vi "Main.vi"(8 "error in (no error)":errorcluster, 11 "TomoBase in":refnum<class "Tomo.lvclass">) -> (0 "error out":errorcluster, 3 "component":refnum<class "Tomo.lvclass">)   [LabVIEW 2012, in "Tomo.lvclass"]
doc: "Main VI of the component."
uses:
  Tomo.lvclass
  <vilib>/Distrio/Murmex/Murmex/command_enum.ctl
  volume map.ctl
  Tomo.lvclass/Tomo.ctl
  <vilib>/Distrio/Murmex/InitialiseMessage/InitialiseMessage.lvclass
  <vilib>/Distrio/Murmex/TerminateMessage/TerminateMessage.lvclass
  <vilib>/Distrio/Murmex/ConfigureMessage/ConfigureMessage.lvclass
  <vilib>/Distrio/Murmex/Murmex/update_cluster.ctl
  <vilib>/Distrio/Murmex/StopMessage/StopMessage.lvclass
  <vilib>/Distrio/Murmex/GenericMessage/GenericMessage.lvclass
  <vilib>/Distrio/Murmex/Murmex/Set configure at initialise.vi
  <vilib>/Distrio/Murmex/Murmex/Set log reference.vi
  <vilib>/Distrio/Murmex/Murmex/Set VI reference.vi
  <vilib>/Distrio/Murmex/Murmex/Set write log to disk.vi
  <vilib>/Distrio/Murmex/Message/Add or replace parameter.vi
  <vilib>/Distrio/Murmex/Murmex/Murmex.lvclass
  <vilib>/Distrio/Murmex/Message/Message.lvclass
panel:
  in  "Tab Control":T1(tab)
  in  "Volume map":T2
  out "TB":dbl format="%#_2g"
  out "Tomography progress":dbl(slide) scale=0.0..1.0
  in  "experiment name":string
  in  "Z step size":dbl[unit]=1e-06
  in  "X step size":dbl[unit]=0.0005
  in  "Y step size":dbl[unit]=0.0005
  in  "Timelapse stacks":dbl=1.0
  in  "starting angle":dbl[unit]
  in  "button::start":bool
  out "Estimated remaining time":dbl format="- %<%H:%M:%S>t"
  in  "X min":dbl[unit]
  in  "X max":dbl[unit]
  in  "Y min":dbl[unit]
  in  "Y max":dbl[unit]
  in  "Z min":dbl[unit]
  in  "Z max":dbl[unit]
  in  "Pre tomo volume file":path
  in  "Pre tomo binary images path":path
  in  "button::pretomo calc":bool
  in  "Custom volume path":path
  in  "Experimenter email address":string
  in  "Experimenter name":string
  in  "generic command":string
  in  "button::send command":bool
  out "log":string
  in  "ID":string="tomo"
  in  "command":T3
  in  "recipient":string
  in  "button::configure":bool
  in  "button::quit":bool
  in  "terminate?":bool
  # "Tomo\n\nImplemented by:\nLudovico Silvestri\nUniversity of Florence, Italy"
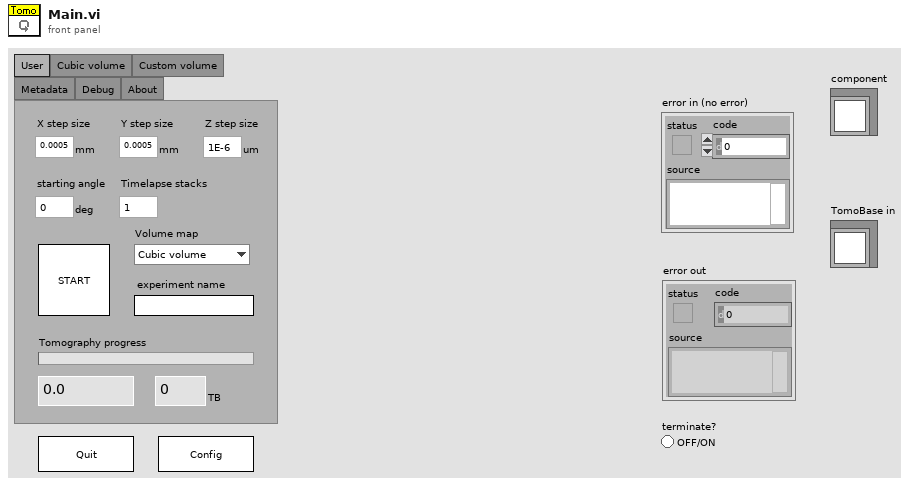
[diagram p1: front panel]
types:
  T1 = enum32{"User", "Cubic volume", "Custom volume", "Metadata", "Debug", "About"}
  T2 = typedef "Tomo.lvclass/volume map.ctl" = enum16{"Cubic volume", "Custom volume", "Self-generate volume", "Time- tomography"}
  T3 = typedef "Murmex.lvlib/Murmex.lvclass/command_enum.ctl" = enum16{"null", "initialise", "reset", "terminate", "acknowledge", "update", "inspect", "inform", "proceed", "start", "stop", "fetch", "configure", "generic"}
  T4 = enum32{"Page Enabled", "Page Disabled", "Page Disabled & Grayed"}
  T5 = typedef "Murmex.lvlib/Murmex.lvclass/update_cluster.ctl" = cluster{"target ID":string, "key chains":string[], "values":variant[]}
  T6 = enum8{"Enabled", "Disabled", "Disabled and Grayed Out"}
  T7 = enum16{"Cubic volume", "Custom volume", "Self-generate volume"}
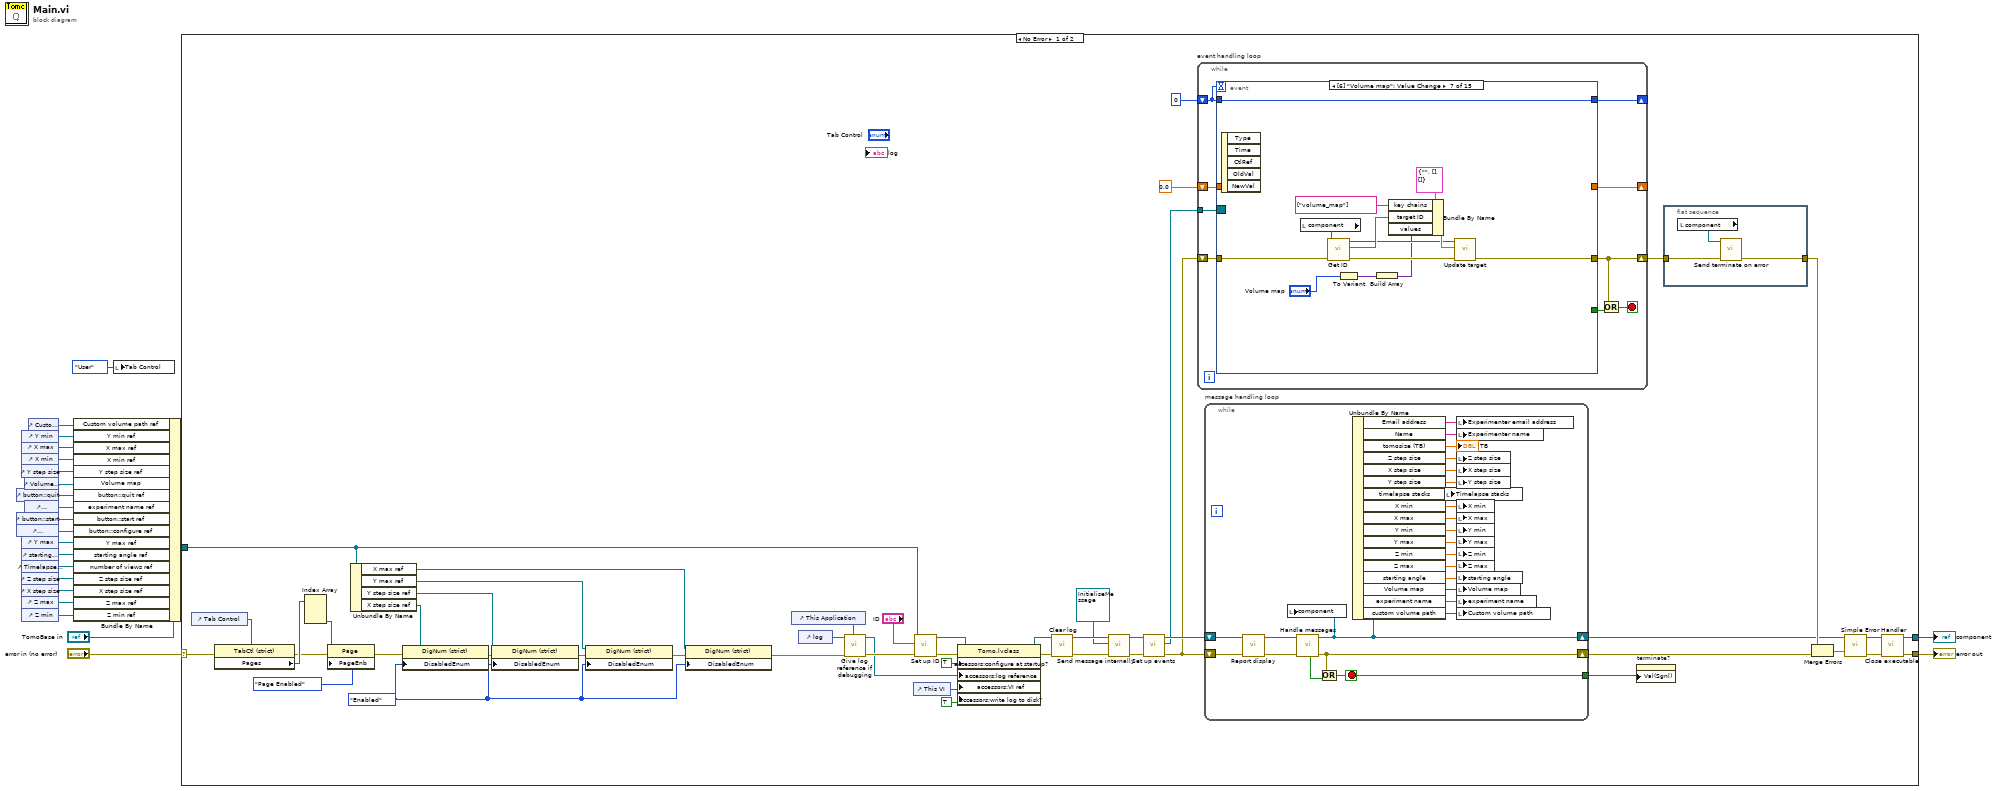
[diagram p0: block diagram]
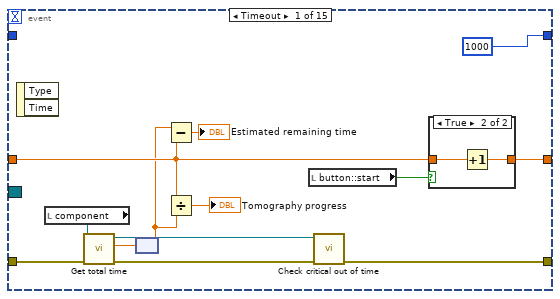
[diagram p2: hidden frame]
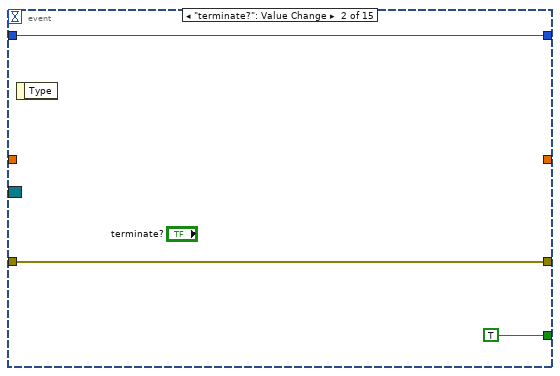
[diagram p4: hidden frame]
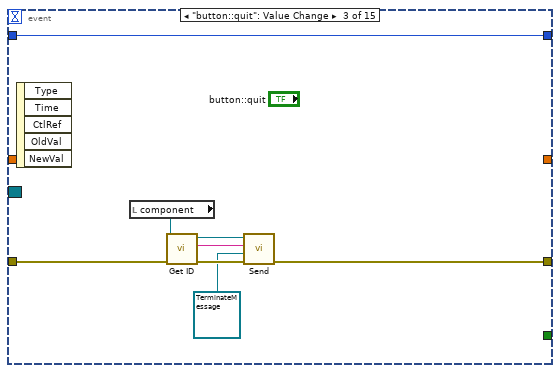
[diagram p5: hidden frame]
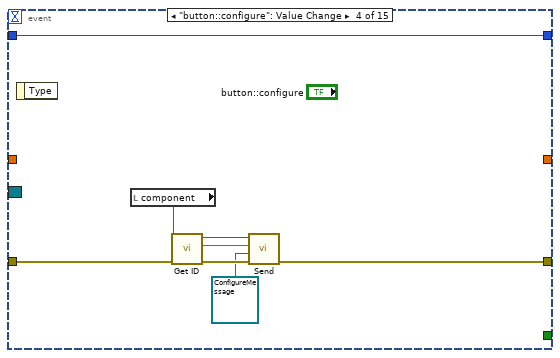
[diagram p6: hidden frame]
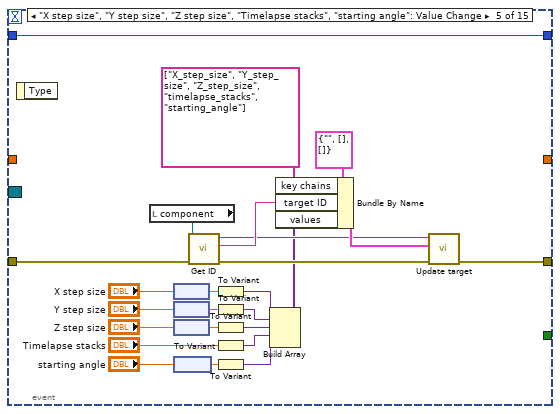
[diagram p7: hidden frame]
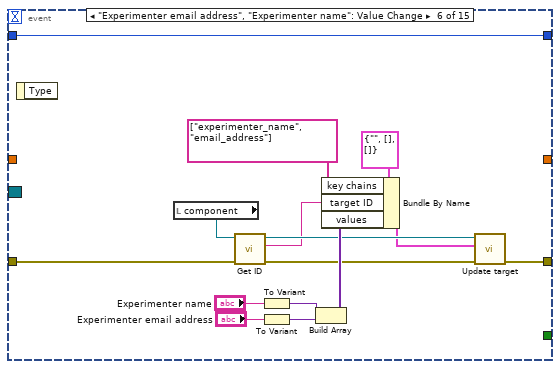
[diagram p8: hidden frame]
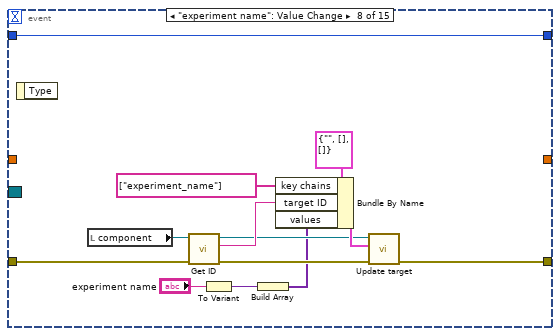
[diagram p9: hidden frame]
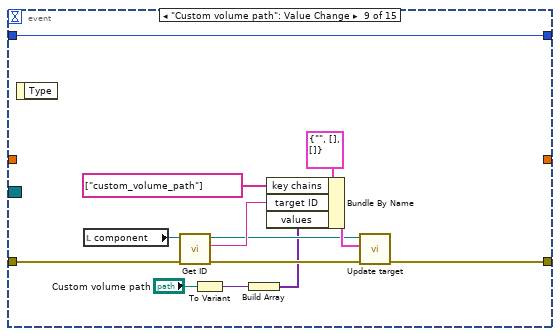
[diagram p10: hidden frame]
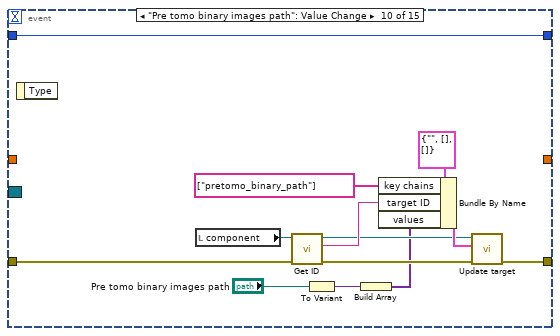
[diagram p11: hidden frame]
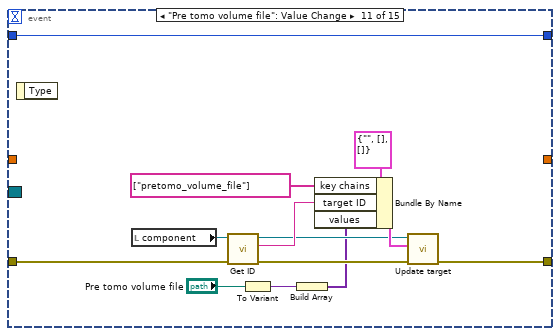
[diagram p12: hidden frame]
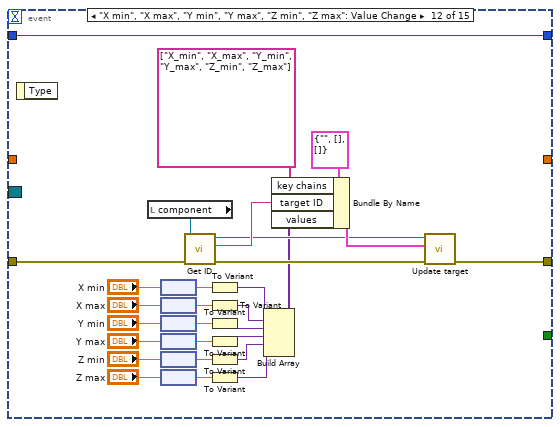
[diagram p13: hidden frame]
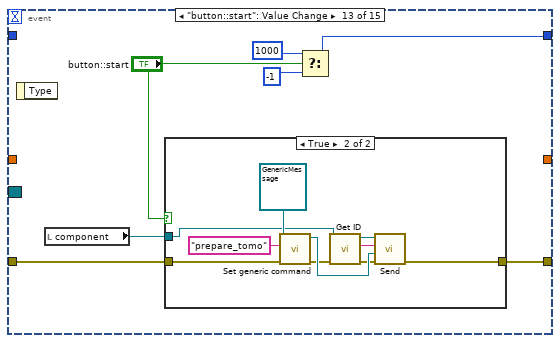
[diagram p14: hidden frame]
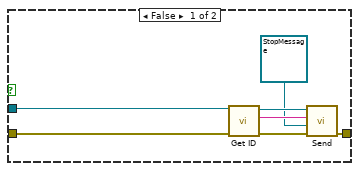
[diagram p15: hidden frame]
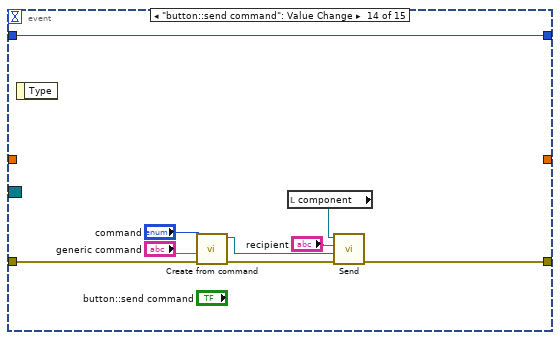
[diagram p16: hidden frame]
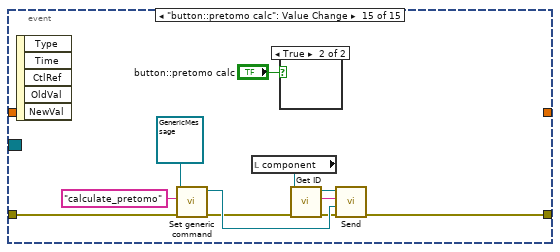
[diagram p17: hidden frame]
diagram:
  n1 = control-ref of="button::quit"() -> (w13:refnum<vi>)
  n2 = control-ref of="button::start"() -> (w11:refnum<vi>)
  n3 = control-ref of="button::configure"() -> (w10:refnum<vi>)
  n4 = control-ref of="Y min"() -> (w17:refnum<vi>)
  n5 = control-ref of="X max"() -> (w16:refnum<vi>)
  n6 = control-ref of="X min"() -> (w15:refnum<vi>)
  n7 = control-ref of="Y step size"() -> (w14:refnum<vi>)
  n8 = control-ref of="Y max"() -> (w9:refnum<vi>)
  n9 = control-ref of="starting angle"() -> (w8:refnum<vi>)
  n10 = control-ref of="Timelapse stacks"() -> (w7:refnum<vi>)
  n11 = control-ref of="Z step size"() -> (w6:refnum<vi>)
  n12 = control-ref of="X step size"() -> (w5:refnum<vi>)
  n13 = control-ref of="Z max"() -> (w4:refnum<vi>)
  n14 = control-ref of="Z min"() -> (w3:refnum<vi>)
  n15 = control-ref of="Volume map"() -> (w1:refnum<vi>)
  n16 = control-ref of="experiment name"() -> (w12:refnum<vi>)
  n17 = control-ref of="Custom volume path"() -> (w18:refnum<vi>)
  n18 = Bundle By Name(cluster="TomoBase in", "Custom volume path ref"=w18, "Y min ref"=w17, "X max ref"=w16, "X min ref"=w15, "Y step size ref"=w14, "Volume map"=w1, "button::quit ref"=w13, "experiment name ref"=w12, "button::start ref"=w11, "button::configure ref"=w10, "Y max ref"=w9, "starting angle ref"=w8, "number of views ref"=w7, "Z step size ref"=w6, "X step size ref"=w5, "Z max ref"=w4, "Z min ref"=w3) -> (w19:refnum<class "Tomo.lvclass">)
  n19 = local write "Tab Control"(T1."User" ("Tab Control")) -> ()
  n20 = case shown="No Error" "error in (no error)" {
    selector: "error in (no error)" -> [w40 w322]
    tunnel: w19 -> [w34 w321]
    tunnel: [w49 w322] -> w22
    tunnel: [w47 w321] -> w21
    frame No Error {
      w24 = T6."Enabled" ("Disabled")
      n21 = control-ref of="Tab Control"() -> (w39:refnum<vi>)
      n22 = property class="TabCtl (strict)"(reference=w39, error in=w40) -> (error out=w37:errorcluster, "Pages"=w38:refnum<vi>[])  [unwired: 1 out]
      n23 = Index Array(array=w38) -> (element #3=w36:refnum<vi>)  [unwired: 3 in, 2 out]
      n24 = property class="Page"(reference=w36, error in=w37, "PageEnb"=T4."Page Enabled" ("Page Enabled State")) -> (error out=w33:errorcluster)  [unwired: 1 out]
      n25 = Unbundle By Name(w34) -> ("X max ref"=w25:refnum<vi>, "Y max ref"=w26:refnum<vi>, "Y step size ref"=w27:refnum<vi>, "X step size ref"=w28:refnum<vi>)
      n26 = property class="DigNum (strict)"(reference=w28, error in=w33, "DisabledEnum"=w24) -> (error out=w32:errorcluster)  [unwired: 1 out]
      n27 = property class="DigNum (strict)"(reference=w27, error in=w32, "DisabledEnum"=w24) -> (error out=w31:errorcluster)  [unwired: 1 out]
      n28 = property class="DigNum (strict)"(reference=w26, error in=w31, "DisabledEnum"=w24) -> (error out=w30:errorcluster)  [unwired: 1 out]
      n29 = property class="DigNum (strict)"(reference=w25, error in=w30, "DisabledEnum"=w24) -> (error out=w29:errorcluster)  [unwired: 1 out]
      n30 = control-ref of="This Application"() -> (w42:refnum<vi>)
      n31 = control-ref of="log"() -> (w44:refnum<vi>)
      n32 = call "Give log reference if debugging.vi"("application ref"=w42, "error in (no error)"=w29, "log reference in"=w44) -> ("error out"=w45:errorcluster, "log reference out"=w43:refnum<vi>)  [unwired: 6 in, 1 out]
      n33 = control-ref of="This VI"() -> (w70:refnum<vi>)
      n34 = call <vilib>:"Set up ID.vi"("error in (no error)"=w45, "component ID"="ID", "MurmexBase in"=w34) -> ("error out"=w69:errorcluster, "MurmexBase out"=w67:refnum<class "Tomo.lvclass">)  [unwired: 6 in, 1 out]
      n35 = property class="Tomo.lvclass"(reference=w67, error in=w69, "accessors:configure at startup?"=TRUE ("configure at startup?"), "accessors:log reference"=w43, "accessors:VI ref"=w70, "accessors:write log to disk?"=TRUE ("write log to disk?")) -> (reference out=w65:refnum<class "Tomo.lvclass">, error out=w66:errorcluster)
      n36 = call <vilib>:"Clear log.vi"("error in (no error)"=w66, "MurmexBase in"=w65) -> ("error out"=w64:errorcluster, "MurmexBase out"=w63:refnum<class "Tomo.lvclass">)  [unwired: 8 in]
      n37 = call <vilib>:"Send message internally.vi"("error in (no error)"=w64, "Message"=refnum<class "InitialiseMessage.lvclass"> refnum ("Message in"), "Murmex in"=w63) -> ("error out"=w61:errorcluster, "Murmex out"=w60:refnum<class "Tomo.lvclass">)  [unwired: 7 in]
      n38 = call <vilib>:"Set up events.vi"("error in (no error)"=w61, "MurmexBase in"=w60) -> ("error out"=w58:errorcluster, "Event Registration Refnum"=w57:refnum<event-registration>, "MurmexBase out"=w59:refnum<class "Tomo.lvclass">)  [unwired: 7 in]
      n39 = while "event handling loop" {
        shift-right: [w78] -> w55
        shift-left: w58 -> [w83]
        tunnel: w57 -> [w82]
        shift-right: [w80] -> _
        shift-left: 0 -> [w81]
        shift-right: [w75] -> _
        shift-left: 0.0 -> [w76]
        stop <- w77 stop-if-true
        n40 = event shown="[6] \"Volume map\": Value Change" {
          selector: w82 -> [_ _ _ _ _ _ _ _ _ _ _ _ _ _ _]
          dyn-events: _ -> [_ _ _ _ _ _ _ _ _ _ _ _ _ _ _]
          timeout: w81 -> [_ _ _ _ _ _ _ _ _ _ _ _ _ _ _]
          tunnel: [w85 w100 w107 w113 w141 w149 w165 w173 w189 w202 w215 w246 w258 w277 w286] -> w78
          tunnel: w83 -> [w96 w100 w109 w114 w139 w148 w167 w176 w188 w201 w214 w244 w257 w283 w287]
          tunnel: w81 -> [_ w99 w102 w110 w122 w143 w164 w172 w184 w198 w211 w230 _ w276 _]
          tunnel: [1000 w99 w102 w110 w122 w143 w164 w172 w184 w198 w211 w230 w252 w276 _] -> w80
          tunnel: [_ TRUE _ _ _ _ _ _ _ _ _ _ _ _ _] -> w79
          tunnel: w76 -> [w94 _ _ _ _ _ _ _ _ _ _ _ _ _ _]
          tunnel: [w93 _ _ _ _ _ _ _ _ _ _ _ _ _ _] -> w75
          event Timeout {
            n41 = event-data() -> ()  [unwired: 1 in, 2 out]
            n42 = local read "component"() -> (w92:refnum<class "Tomo.lvclass">)
            n43 = call-dynamic "Get total time.vi"("error in (no error)"=w96, "Tomo in"=w92) -> ("error out"=w95:errorcluster, "Total time"=w91:dbl[unit], "Tomo out"=w84:refnum<class "Tomo.lvclass">)  [unwired: 7 in]
            n44 = node(w91) -> (w89:dbl)
            n45 = Subtract(x=w89, y=w94) -> (x-y=→"Estimated remaining time":dbl)
            n46 = Divide(x=w94, y=w89) -> (x/y=→"Tomography progress":dbl)
            n47 = local read "button::start"() -> (w86:bool)
            n48 = call-dynamic "Check critical out of time.vi"("error in (no error)"=w95, "Tomo in"=w84) -> ("error out"=w85:errorcluster)  [unwired: 8 in, 1 out]
            n49 = case shown="True" w86 {
              tunnel: w94 -> [_ w98]
              tunnel: [_ w97] -> w93
              frame False {
              }
              frame True {
                n50 = Increment(x=w98) -> (x+1=w97:dbl)
              }
            }
          }
          event "terminate?": Value Change {
            n51 = event-data() -> ()  [unwired: 1 in, 1 out]
          }
          event "button::quit": Value Change {
            n52 = event-data() -> ()  [unwired: 1 in, 5 out]
            n53 = local read "component"() -> (w106:refnum<class "Tomo.lvclass">)
            n54 = call <vilib>:"Get ID.vi"("error in (no error)"=w109, "Murmex in"=w106) -> ("error out"=w108:errorcluster, "component id"=w104:string, "Murmex out"=w105:refnum<class "Tomo.lvclass">)  [unwired: 7 in]
            n55 = call <vilib>:"Send.vi"("error in (no error)"=w108, "Message"=refnum<class "TerminateMessage.lvclass"> refnum ("Distrio Murmex 1.1:TerminateMessage"), "recipient"=w104, "Murmex in"=w105) -> ("error out"=w107:errorcluster)  [unwired: 6 in, 1 out]
          }
          event "button::configure": Value Change {
            n56 = event-data() -> ()  [unwired: 1 in, 1 out]
            n57 = local read "component"() -> (w112:refnum<class "Tomo.lvclass">)
            n58 = call <vilib>:"Get ID.vi"("error in (no error)"=w114, "Murmex in"=w112) -> ("error out"=w117:errorcluster, "component id"=w115:string, "Murmex out"=w116:refnum<class "Tomo.lvclass">)  [unwired: 7 in]
            n59 = call <vilib>:"Send.vi"("error in (no error)"=w117, "Message"=refnum<class "ConfigureMessage.lvclass"> refnum ("Distrio Murmex 1.1:ConfigureMessage"), "recipient"=w115, "Murmex in"=w116) -> ("error out"=w113:errorcluster)  [unwired: 6 in, 1 out]
          }
          event "X step size", "Y step size", "Z step size", "Timelapse stacks", "starting angle": Value Change {
            n60 = event-data() -> ()  [unwired: 1 in, 1 out]
            n61 = local read "component"() -> (w137:refnum<class "Tomo.lvclass">)
            n62 = node("X step size") -> (w121:dbl)
            n63 = node("Y step size") -> (w120:dbl)
            n64 = node("Z step size") -> (w119:dbl)
            n65 = node("starting angle") -> (w118:dbl)
            n66 = call <vilib>:"Get ID.vi"("error in (no error)"=w139, "Murmex in"=w137) -> ("error out"=w140:errorcluster, "component id"=w138:string, "Murmex out"=w135:refnum<class "Tomo.lvclass">)  [unwired: 7 in]
            n67 = To Variant(anything=w121) -> (Variant=w125:variant)
            n68 = To Variant(anything=w120) -> (Variant=w126:variant)
            n69 = To Variant(anything=w119) -> (Variant=w129:variant)
            n70 = To Variant(anything="Timelapse stacks") -> (Variant=w128:variant)
            n71 = To Variant(anything=w118) -> (Variant=w127:variant)
            n72 = Build Array(w125, w126, w129, w128, w127) -> (w124:variant[])
            n73 = Bundle By Name(cluster=T5 {"target ID"="", "key chains"=[], "values"=[]} ("update cluster"), "key chains"=string[] ["X_step_size", "Y_step_size", "Z_step_size", "timelapse_stacks", "starting_angle"], "target ID"=w138, "values"=w124) -> (w136:T5)
            n74 = call <vilib>:"Update target.vi"("error in (no error)"=w140, "update cluster"=w136, "MurmexBase in"=w135) -> ("error out"=w141:errorcluster)  [unwired: 7 in, 1 out]
          }
          event "Experimenter email address", "Experimenter name": Value Change {
            n75 = event-data() -> ()  [unwired: 1 in, 1 out]
            n76 = local read "component"() -> (w144:refnum<class "Tomo.lvclass">)
            n77 = call <vilib>:"Get ID.vi"("error in (no error)"=w148, "Murmex in"=w144) -> ("error out"=w151:errorcluster, "component id"=w152:string, "Murmex out"=w154:refnum<class "Tomo.lvclass">)  [unwired: 7 in]
            n78 = To Variant(anything="Experimenter name") -> (Variant=w156:variant)
            n79 = To Variant(anything="Experimenter email address") -> (Variant=w155:variant)
            n80 = Build Array(w156, w155) -> (w157:variant[])
            n81 = Bundle By Name(cluster=T5 {"target ID"="", "key chains"=[], "values"=[]} ("update cluster"), "key chains"=string[] ["experimenter_name", "email_address"], "target ID"=w152, "values"=w157) -> (w153:T5)
            n82 = call <vilib>:"Update target.vi"("error in (no error)"=w151, "update cluster"=w153, "MurmexBase in"=w154) -> ("error out"=w149:errorcluster)  [unwired: 7 in, 1 out]
          }
          event Value Change {
            n83 = event-data() -> ()  [unwired: 1 in, 5 out]
            n84 = local read "component"() -> (w159:refnum<class "Tomo.lvclass">)
            n85 = call <vilib>:"Get ID.vi"("error in (no error)"=w167, "Murmex in"=w159) -> ("error out"=w166:errorcluster, "component id"=w170:string, "Murmex out"=w168:refnum<class "Tomo.lvclass">)  [unwired: 7 in]
            n86 = To Variant(anything="Volume map") -> (Variant=w163:variant)
            n87 = Build Array(w163) -> (w162:variant[])
            n88 = Bundle By Name(cluster=T5 {"target ID"="", "key chains"=[], "values"=[]} ("update cluster"), "key chains"=string[] ["volume_map"], "target ID"=w170, "values"=w162) -> (w169:T5)
            n89 = call <vilib>:"Update target.vi"("error in (no error)"=w166, "update cluster"=w169, "MurmexBase in"=w168) -> ("error out"=w165:errorcluster)  [unwired: 7 in, 1 out]
          }
          event "experiment name": Value Change {
            n90 = event-data() -> ()  [unwired: 1 in, 1 out]
            n91 = local read "component"() -> (w171:refnum<class "Tomo.lvclass">)
            n92 = call <vilib>:"Get ID.vi"("error in (no error)"=w176, "Murmex in"=w171) -> ("error out"=w180:errorcluster, "component id"=w183:string, "Murmex out"=w181:refnum<class "Tomo.lvclass">)  [unwired: 7 in]
            n93 = To Variant(anything="experiment name") -> (Variant=w179:variant)
            n94 = Build Array(w179) -> (w178:variant[])
            n95 = Bundle By Name(cluster=T5 {"target ID"="", "key chains"=[], "values"=[]} ("update cluster"), "key chains"=string[] ["experiment_name"], "target ID"=w183, "values"=w178) -> (w182:T5)
            n96 = call <vilib>:"Update target.vi"("error in (no error)"=w180, "update cluster"=w182, "MurmexBase in"=w181) -> ("error out"=w173:errorcluster)  [unwired: 7 in, 1 out]
          }
          event "Custom volume path": Value Change {
            n97 = event-data() -> ()  [unwired: 1 in, 1 out]
            n98 = local read "component"() -> (w186:refnum<class "Tomo.lvclass">)
            n99 = call <vilib>:"Get ID.vi"("error in (no error)"=w188, "Murmex in"=w186) -> ("error out"=w193:errorcluster, "component id"=w196:string, "Murmex out"=w194:refnum<class "Tomo.lvclass">)  [unwired: 7 in]
            n100 = To Variant(anything="Custom volume path") -> (Variant=w192:variant)
            n101 = Build Array(w192) -> (w191:variant[])
            n102 = Bundle By Name(cluster=T5 {"target ID"="", "key chains"=[], "values"=[]} ("update cluster"), "key chains"=string[] ["custom_volume_path"], "target ID"=w196, "values"=w191) -> (w195:T5)
            n103 = call <vilib>:"Update target.vi"("error in (no error)"=w193, "update cluster"=w195, "MurmexBase in"=w194) -> ("error out"=w189:errorcluster)  [unwired: 7 in, 1 out]
          }
          event "Pre tomo binary images path": Value Change {
            n104 = event-data() -> ()  [unwired: 1 in, 1 out]
            n105 = local read "component"() -> (w200:refnum<class "Tomo.lvclass">)
            n106 = call <vilib>:"Get ID.vi"("error in (no error)"=w201, "Murmex in"=w200) -> ("error out"=w206:errorcluster, "component id"=w209:string, "Murmex out"=w207:refnum<class "Tomo.lvclass">)  [unwired: 7 in]
            n107 = To Variant(anything="Pre tomo binary images path") -> (Variant=w205:variant)
            n108 = Build Array(w205) -> (w204:variant[])
            n109 = Bundle By Name(cluster=T5 {"target ID"="", "key chains"=[], "values"=[]} ("update cluster"), "key chains"=string[] ["pretomo_binary_path"], "target ID"=w209, "values"=w204) -> (w208:T5)
            n110 = call <vilib>:"Update target.vi"("error in (no error)"=w206, "update cluster"=w208, "MurmexBase in"=w207) -> ("error out"=w202:errorcluster)  [unwired: 7 in, 1 out]
          }
          event "Pre tomo volume file": Value Change {
            n111 = event-data() -> ()  [unwired: 1 in, 1 out]
            n112 = local read "component"() -> (w213:refnum<class "Tomo.lvclass">)
            n113 = call <vilib>:"Get ID.vi"("error in (no error)"=w214, "Murmex in"=w213) -> ("error out"=w219:errorcluster, "component id"=w222:string, "Murmex out"=w220:refnum<class "Tomo.lvclass">)  [unwired: 7 in]
            n114 = To Variant(anything="Pre tomo volume file") -> (Variant=w218:variant)
            n115 = Build Array(w218) -> (w217:variant[])
            n116 = Bundle By Name(cluster=T5 {"target ID"="", "key chains"=[], "values"=[]} ("update cluster"), "key chains"=string[] ["pretomo_volume_file"], "target ID"=w222, "values"=w217) -> (w221:T5)
            n117 = call <vilib>:"Update target.vi"("error in (no error)"=w219, "update cluster"=w221, "MurmexBase in"=w220) -> ("error out"=w215:errorcluster)  [unwired: 7 in, 1 out]
          }
          event "X min", "X max", "Y min", "Y max", "Z min", "Z max": Value Change {
            n118 = event-data() -> ()  [unwired: 1 in, 1 out]
            n119 = local read "component"() -> (w243:refnum<class "Tomo.lvclass">)
            n120 = node("X min") -> (w229:dbl)
            n121 = node("X max") -> (w228:dbl)
            n122 = node("Y min") -> (w227:dbl)
            n123 = node("Y max") -> (w226:dbl)
            n124 = node("Z min") -> (w224:dbl)
            n125 = node("Z max") -> (w223:dbl)
            n126 = call <vilib>:"Get ID.vi"("error in (no error)"=w244, "Murmex in"=w243) -> ("error out"=w245:errorcluster, "component id"=w250:string, "Murmex out"=w248:refnum<class "Tomo.lvclass">)  [unwired: 7 in]
            n127 = To Variant(anything=w229) -> (Variant=w239:variant)
            n128 = To Variant(anything=w228) -> (Variant=w240:variant)
            n129 = To Variant(anything=w227) -> (Variant=w242:variant)
            n130 = To Variant(anything=w226) -> (Variant=w241:variant)
            n131 = To Variant(anything=w224) -> (Variant=w232:variant)
            n132 = To Variant(anything=w223) -> (Variant=w231:variant)
            n133 = Build Array(w239, w240, w242, w241, w232, w231) -> (w238:variant[])
            n134 = Bundle By Name(cluster=T5 {"target ID"="", "key chains"=[], "values"=[]} ("update cluster"), "key chains"=string[] ["X_min", "X_max", "Y_min", "Y_max", "Z_min", "Z_max"], "target ID"=w250, "values"=w238) -> (w249:T5)
            n135 = call <vilib>:"Update target.vi"("error in (no error)"=w245, "update cluster"=w249, "MurmexBase in"=w248) -> ("error out"=w246:errorcluster)  [unwired: 7 in, 1 out]
          }
          event "button::start": Value Change {
            n136 = event-data() -> ()  [unwired: 1 in, 1 out]
            n137 = local read "component"() -> (w256:refnum<class "Tomo.lvclass">)
            n138 = case shown="True" "button::start" {
              tunnel: [w263 w266] -> w258
              tunnel: w257 -> [w261 w268]
              tunnel: w256 -> [w259 w267]
              frame False {
                n139 = call <vilib>:"Get ID.vi"("error in (no error)"=w261, "Murmex in"=w259) -> ("error out"=w262:errorcluster, "component id"=w264:string, "Murmex out"=w265:refnum<class "Tomo.lvclass">)  [unwired: 7 in]
                n140 = call <vilib>:"Send.vi"("error in (no error)"=w262, "Message"=refnum<class "StopMessage.lvclass"> refnum ("Distrio Murmex 1.1:StopMessage"), "recipient"=w264, "Murmex in"=w265) -> ("error out"=w263:errorcluster)  [unwired: 6 in, 1 out]
              }
              frame True {
                n141 = call <vilib>:"Set generic command.vi"("error in (no error)"=w268, "generic command"="prepare_tomo", "GenericMessage in"=refnum<class "GenericMessage.lvclass"> refnum ("Message in")) -> ("error out"=w270:errorcluster, "GenericMessage out"=w274:refnum<class "GenericMessage.lvclass">)  [unwired: 7 in]
                n142 = call <vilib>:"Get ID.vi"("error in (no error)"=w270, "Murmex in"=w267) -> ("error out"=w271:errorcluster, "component id"=w273:string, "Murmex out"=w272:refnum<class "Tomo.lvclass">)  [unwired: 7 in]
                n143 = call <vilib>:"Send.vi"("error in (no error)"=w271, "Message"=w274, "recipient"=w273, "Murmex in"=w272) -> ("error out"=w266:errorcluster)  [unwired: 6 in, 1 out]
              }
            }
            n144 = Select(t=1000, s="button::start", f=-1) -> (s? t:f=w252:i32)
          }
          event "button::send command": Value Change {
            n145 = event-data() -> ()  [unwired: 1 in, 1 out]
            n146 = call <vilib>:"Create from command.vi"("error in (no error)"=w283, "generic command"="generic command", "command"="command") -> ("error out"=w278:errorcluster, "Message out"=w279:refnum<class "Message.lvclass">)  [unwired: 7 in]
            n147 = local read "component"() -> (w280:refnum<class "Tomo.lvclass">)
            n148 = call <vilib>:"Send.vi"("error in (no error)"=w278, "Message"=w279, "recipient"="recipient", "Murmex in"=w280) -> ("error out"=w277:errorcluster)  [unwired: 6 in, 1 out]
          }
          event "button::pretomo calc": Value Change {
            n149 = event-data() -> ()  [unwired: 1 in, 5 out]
            n150 = call <vilib>:"Set generic command.vi"("error in (no error)"=w287, "generic command"="calculate_pretomo", "GenericMessage in"=refnum<class "GenericMessage.lvclass"> refnum ("Message in")) -> ("error out"=w289:errorcluster, "GenericMessage out"=w293:refnum<class "GenericMessage.lvclass">)  [unwired: 7 in]
            n151 = local read "component"() -> (w285:refnum<class "Tomo.lvclass">)
            n152 = case shown="True" "button::pretomo calc" {
              frame False {
              }
              frame True {
              }
            }
            n153 = call <vilib>:"Get ID.vi"("error in (no error)"=w289, "Murmex in"=w285) -> ("error out"=w290:errorcluster, "component id"=w292:string, "Murmex out"=w291:refnum<class "Tomo.lvclass">)  [unwired: 7 in]
            n154 = call <vilib>:"Send.vi"("error in (no error)"=w290, "Message"=w293, "recipient"=w292, "Murmex in"=w291) -> ("error out"=w286:errorcluster)  [unwired: 6 in, 1 out]
          }
        }
        n155 = Or(x=w78, y=w79) -> (x .or. y?=w77:bool)
      }
      n156 = while "message handling loop" {
        shift-right: [w301] -> w54
        shift-left: w58 -> [w299]
        shift-right: [w300] -> w48
        shift-left: w59 -> [w297]
        tunnel: [w319] -> w50
        stop <- w319 stop-if-true
        n157 = call-dynamic "Report display.vi"("error in (no error)"=w299, "Tomo in"=w297) -> ("error out"=w298:errorcluster, "Tomo out"=w296:refnum<class "Tomo.lvclass">)  [unwired: 8 in]
        n158 = call <vilib>:"Handle messages.vi"("error in (no error)"=w298, "Murmex in"=w296) -> ("error out"=w301:errorcluster, "Murmex out"=w300:refnum<class "Tomo.lvclass">, "terminated?"=w320:bool)  [unwired: 7 in]
        n159 = local write "component"(w300) -> ()
        n160 = Or(x=w301, y=w320) -> (x .or. y?=w319:bool)
        n161 = Unbundle By Name(w300) -> ("Email address"=w302:string, "Name"=w303:string, "tomosize (TB)"=→"TB":dbl, "Z step size"=w310:dbl[unit], "X step size"=w312:dbl[unit], "Y step size"=w311:dbl[unit], "timelapse stacks"=w309:dbl, "X min"=w318:dbl[unit], "X max"=w317:dbl[unit], "Y min"=w316:dbl[unit], "Y max"=w315:dbl[unit], "Z min"=w314:dbl[unit], "Z max"=w313:dbl[unit], "starting angle"=w308:dbl[unit], "Volume map"=w307:T7, "experiment name"=w306:string, "custom volume path"=w305:path)
        n162 = local write "Timelapse stacks"(w309) -> ()
        n163 = local write "Experimenter email address"(w302) -> ()
        n164 = local write "Experimenter name"(w303) -> ()
        n165 = local write "Z step size"(w310) -> ()
        n166 = local write "X step size"(w312) -> ()
        n167 = local write "Y step size"(w311) -> ()
        n168 = local write "X min"(w318) -> ()
        n169 = local write "X max"(w317) -> ()
        n170 = local write "Y min"(w316) -> ()
        n171 = local write "Y max"(w315) -> ()
        n172 = local write "Z min"(w314) -> ()
        n173 = local write "Z max"(w313) -> ()
        n174 = local write "starting angle"(w308) -> ()
        n175 = local write "Volume map"(w307) -> ()
        n176 = local write "experiment name"(w306) -> ()
        n177 = local write "Custom volume path"(w305) -> ()
      }
      n178 = property on="terminate?" class="Bool (strict)"("Val(Sgnl)"=w50) -> ()  [unwired: 2 in, 2 out]
      n179 = flat-sequence {
        tunnel: w55 -> [w74]
        tunnel: [w72] -> w53
        frame #0 {
          n180 = local read "component"() -> (w73:refnum<class "Tomo.lvclass">)
          n181 = call <vilib>:"Send terminate on error.vi"("error in (no error)"=w74, "Murmex in"=w73) -> ("error out"=w72:errorcluster)  [unwired: 8 in, 1 out]
        }
      }
      n182 = Merge Errors(w53, w54) -> (w52:errorcluster)
      n183 = call <vilib>:"Simple Error Handler.vi"("error in (no error)"=w52) -> ("error out"=w51:errorcluster)  [unwired: 4 in, 4 out]
      n184 = call <vilib>:"Close executable.vi"("error in (no error)"=w51, "MurmexBase in"=w48) -> ("error out"=w49:errorcluster, "MurmexBase out"=w47:refnum<class "Tomo.lvclass">)  [unwired: 8 in]
    }
    frame Error {
    }
  }
  "error out" <- w22
  "component" <- w21
